vi "BUILD_vipb path.vi"() -> (3 "appended path":path)   [LabVIEW 2013]
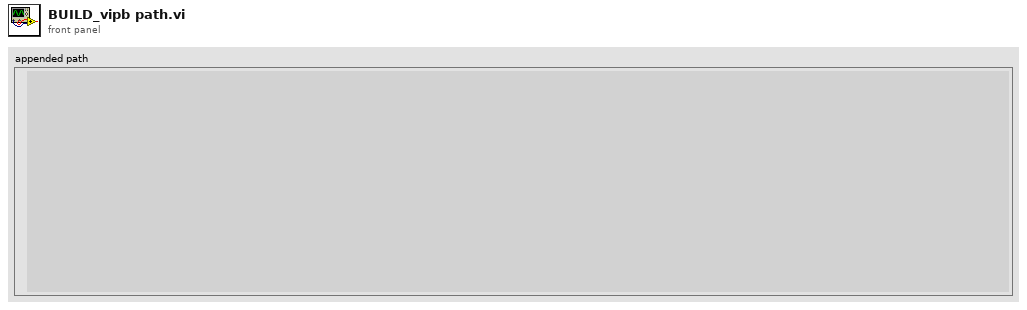
[diagram p1: front panel]
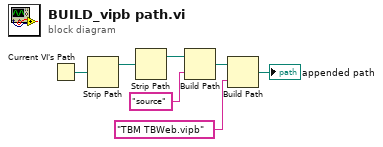
[diagram p0: block diagram]
diagram:
  n1 = Current VI's Path() -> (path=w3:path)
  n2 = Strip Path(path=w3) -> (stripped path=w4:path)  [unwired: 1 out]
  n3 = Strip Path(path=w4) -> (stripped path=w5:path)  [unwired: 1 out]
  n4 = Build Path(base path=w5, name or relative path="source") -> (appended path=w2:path)
  n5 = Build Path(base path=w2, name or relative path="TBM TBWeb.vipb") -> (appended path=→"appended path":path)
